vi "Set lasers power.vi"(0 "Green power (mW)":u16(knob) scale=0.0..1000.0, 1 "Blue power (mW)":u16(knob) scale=0.0..1000.0) -> (2 "Green laser setting error":errorcluster, 3 "Blue laser setting error":errorcluster, 4 "Initialisation error":errorcluster)   [LabVIEW 2014]
uses:
  Laser enum.ctl
  Commands.ctl
panel:
  # "PN 05/11/2014"
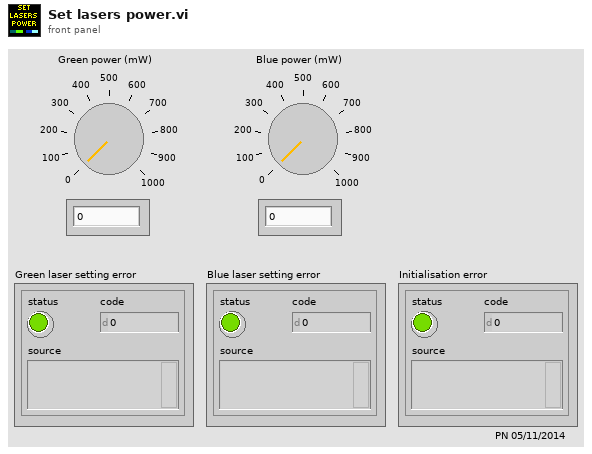
[diagram p1: front panel]
types:
  T1 = typedef "Commands.ctl" = u8
  T2 = typedef "Laser enum.ctl" = u8
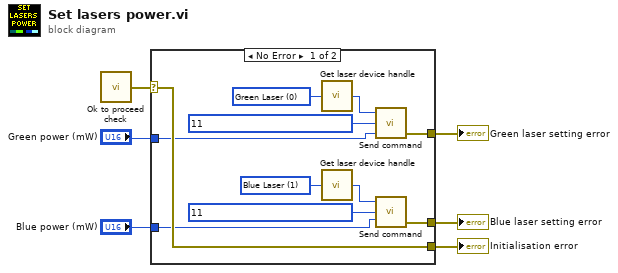
[diagram p0: block diagram]
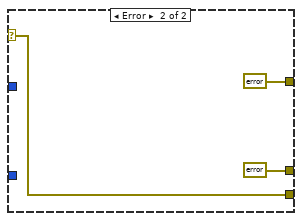
[diagram p2: hidden frame]
diagram:
  n1 = call "Ok to proceed check.vi"() -> ("Error"=w4:errorcluster)
  n2 = case shown="No Error" w4 {
    selector: w4 -> [w17 w20]
    tunnel: [w14 errorcluster {"status"=FALSE, "code"=0, "source"=""} ("Error")] -> w6
    tunnel: [w13 errorcluster {"status"=FALSE, "code"=0, "source"=""} ("Error")] -> w5
    tunnel: [w17 w20] -> w3
    tunnel: "Green power (mW)" -> [w12 _]
    tunnel: "Blue power (mW)" -> [w11 _]
    frame No Error {
      w9 = T2 1 items=["Green Laser", "Blue Laser"] ("Selected laser")
      w10 = T2 0 items=["Green Laser", "Blue Laser"] ("Selected laser")
      n3 = call "Get laser device handle.vi"("Selected laser"=w10) -> ("Device handle"=w7:u32)
      n4 = call "Get laser device handle.vi"("Selected laser"=w9) -> ("Device handle"=w8:u32)
      n5 = call "Send command.vi"("Value"=w12, "Command"=T1 11, "Device handle"=w7) -> ("Error"=w14:errorcluster)  [unwired: 2 out]
      n6 = call "Send command.vi"("Value"=w11, "Command"=T1 11, "Device handle"=w8) -> ("Error"=w13:errorcluster)  [unwired: 2 out]
    }
    frame Error {
    }
  }
  "Green laser setting error" <- w6
  "Blue laser setting error" <- w5
  "Initialisation error" <- w3
